vi "Calibration-LineN-Acquisition.vi"(7 "Cal Line?":i32, 8 "error in (no error)":errorcluster, 11 "Calibration-RunTest in":refnum<class "Calibration-RunTest.lvclass">) -> (0 "error out":errorcluster, 3 "Calibration-RunTest out":refnum<class "Calibration-RunTest.lvclass">)   [LabVIEW 2014, in "Calibration-RunTest.lvclass"]
uses:
  Calibration-RunTest.lvclass
  Reuse Library/Keyence LK-G5000/Public/enum/LKIF_OUTNO.ctl
  Reuse Library/Keyence LK-G5000/Keyence LK-G5000.lvlib
  Motion Control/Motion-ControlAll.lvclass
panel:
  out "Raw Cal Data":dbl[](array[numeric])
  out "Laser Value":sgl format="%_6g"
  out "stop collecting":bool=TRUE
  out "Meas 1 Dyn Data":dbl[](graph)
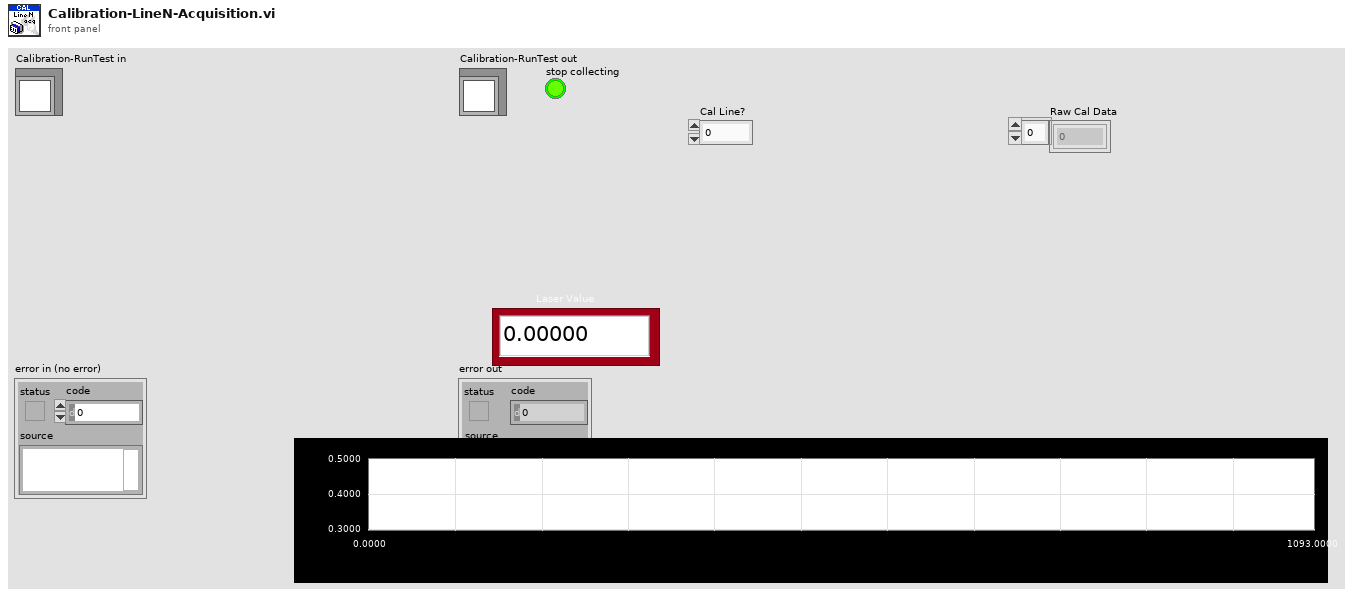
[diagram p1: front panel]
types:
  T1 = typedef "Keyence LK-G5000.lvlib/LKIF_OUTNO.ctl" = i32
  T2 = typedef "Keyence LK-G5000.lvlib/LKIF_FLOATRESULT.ctl" = i32
  T3 = cluster{"OutNo":i32, "LKIF_FLOATRESULT":T2, "Value":sgl}[]
  T4 = cluster{"OutNo":i32, "LKIF_FLOATRESULT":T2, "Value":sgl}
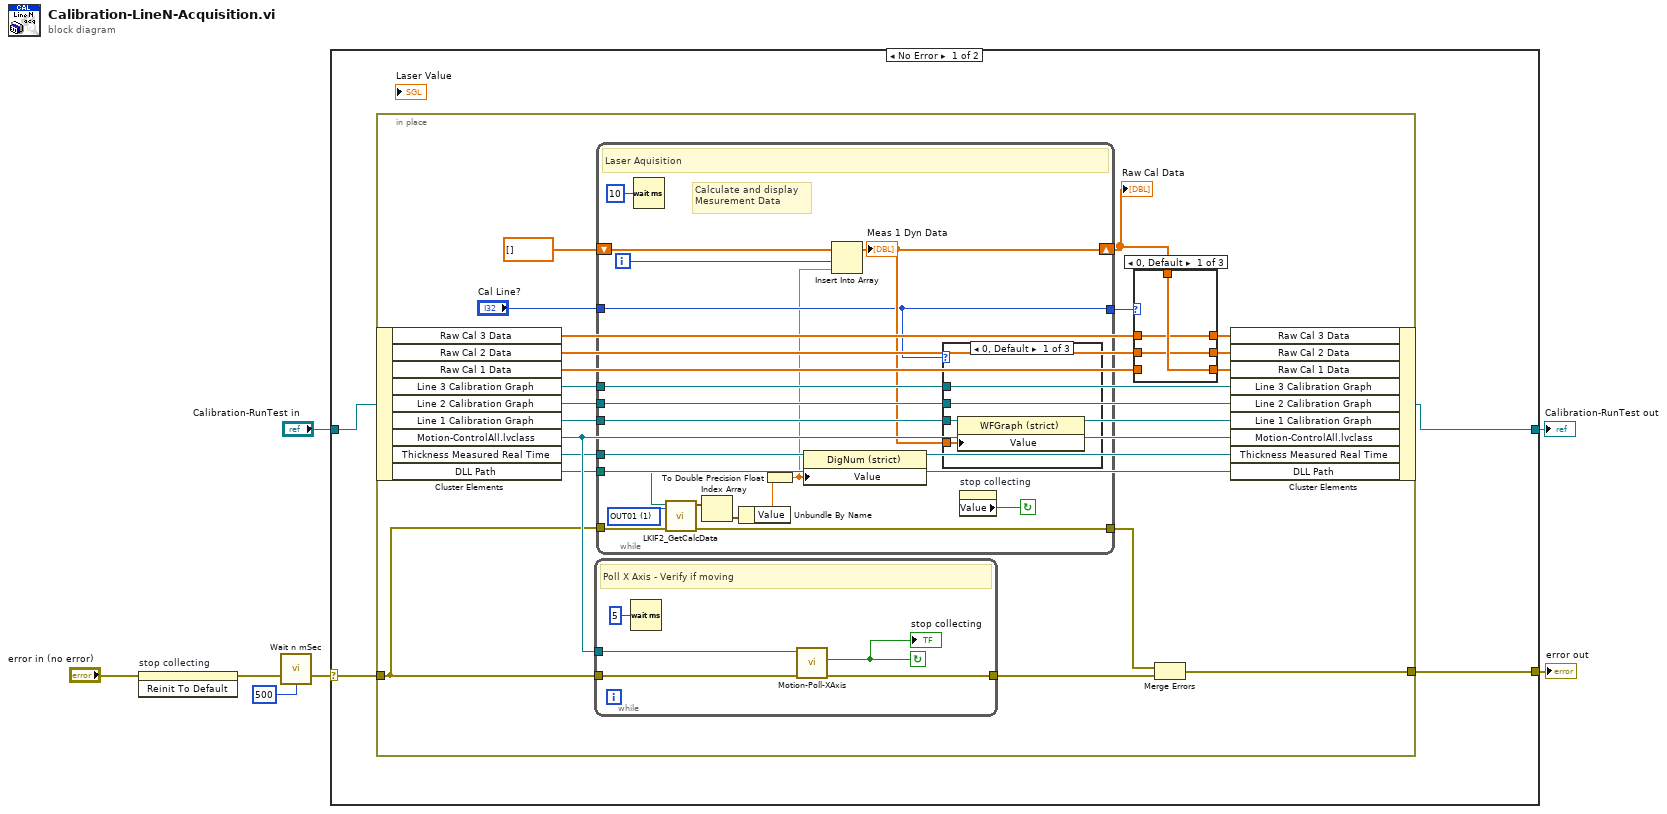
[diagram p0: block diagram]
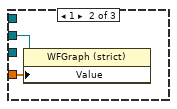
[diagram p4: hidden frame]
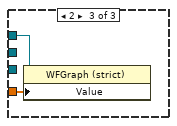
[diagram p5: hidden frame]
diagram:
  n1 = invoke on="stop collecting" class="Bool (strict)" method="Reinit To Default"(error in="error in (no error)") -> (error out=w1:errorcluster)  [unwired: 2 in, 2 out]
  n2 = call <vilib>:"Wait n mSec.vi"("error in (no error)"=w1, "Milliseconds to Wait (500)"=u32 500) -> ("error out"=w2:errorcluster)  [unwired: 13 in]
  n3 = case shown="No Error" w2 {
    selector: w2 -> [w10 w71]
    tunnel: [w9 w71] -> w7
    tunnel: [w8 w70] -> w5
    tunnel: "Calibration-RunTest in" -> [w11 w70]
    frame No Error {
      n4 = in-place {
        in-place-border: w10 -> [w12]
        in-place-border: [w29] -> w9
        n5 = in-place-cluster #1(w11) -> ("Raw Cal 3 Data"=w17:dbl[], "Raw Cal 2 Data"=w19:dbl[], "Raw Cal 1 Data"=w20:dbl[], "Line 3 Calibration Graph"=w25:refnum<vi>, "Line 2 Calibration Graph"=w26:refnum<vi>, "Line 1 Calibration Graph"=w27:refnum<vi>, "Motion-ControlAll.lvclass"=w28:refnum<class "Motion-ControlAll.lvclass">, "Thickness Measured Real Time"=w14:refnum<vi>, "DLL Path"=w13:path)
        n6 = while {
          tunnel: w12 -> [w44]
          tunnel: [w42] -> w31
          tunnel: w28 -> [w43]
          stop <- w41 continue-if-true
          # "Poll X Axis - Verify if moving"
          n7 = Wait (ms)(milliseconds to wait=u32 5) -> ()  [unwired: 1 out]
          n8 = call "Motion-Poll-XAxis.vi"("error in (no error)"=w44, "Motion-ControlAll in"=w43) -> ("error out"=w42:errorcluster, "X axis \nstopped"=w41:bool)  [unwired: 7 in, 1 out]
          "stop collecting" <- w41
        }
        n9 = while {
          tunnel: w12 -> [w63]
          tunnel: [w59] -> w30
          shift-right: [w53] -> w22
          shift-left: dbl[] [] -> [w57]
          tunnel: w27 -> [w54]
          tunnel: w26 -> [w52]
          tunnel: w25 -> [w51]
          tunnel: "Cal Line?" -> [w50]
          tunnel: [w50] -> w23
          tunnel: w14 -> [w49]
          tunnel: w13 -> [w46]
          i -> [w56]
          stop <- w55 continue-if-true
          w62 = T1 1 items=["OUT01"=1, "OUT02"=2, "OUT03"=4, "OUT04"=8, "OUT05"=16, "OUT06"=32, "OUT07"=64, "OUT08"=128, "OUT09"=256, "OUT10"=512, "OUT11"=1024, "OUT12"=2048, "ALL OUT"=4095] ("OutNo (OUT1)")
          # "Calculate and display \nMesurement Data"
          # "Laser Aquisition"
          n10 = Wait (ms)(milliseconds to wait=u32 10) -> ()  [unwired: 1 out]
          n11 = call "LKIF2_GetCalcData.vi"("OutNo (OUT1)"=w62, "error in (no error)"=w63, "path in"=w46) -> ("error out"=w59:errorcluster, "CalcData"=w61:T3)  [unwired: 7 in]
          n12 = Index Array(array=w61) -> (element=w60:T4)  [unwired: 1 in]
          n13 = Unbundle By Name(w60) -> ("Value"=w48:sgl)
          n14 = To Double Precision Float(number=w48) -> (double precision float=w47:dbl)
          n15 = property class="DigNum (strict)"(reference=w49, "Value"=w47) -> ()  [unwired: 1 in, 2 out]
          n16 = Insert Into Array(array=w57, index=w56, new element=w47) -> (w53:dbl[])
          "Meas 1 Dyn Data" <- w53
          n17 = case shown="0, Default" w50 {
            tunnel: w54 -> [w65 _ _]
            tunnel: w53 -> [w64 w66 w69]
            tunnel: w52 -> [_ w67 _]
            tunnel: w51 -> [_ _ w68]
            frame 0, Default {
              n18 = property class="WFGraph (strict)"(reference=w65, "Value"=w64) -> ()  [unwired: 1 in, 2 out]
            }
            frame 1 {
              n19 = property class="WFGraph (strict)"(reference=w67, "Value"=w66) -> ()  [unwired: 1 in, 2 out]
            }
            frame 2 {
              n20 = property class="WFGraph (strict)"(reference=w68, "Value"=w69) -> ()  [unwired: 1 in, 2 out]
            }
          }
          n21 = property on="stop collecting" class="Bool (strict)"() -> ("Value"=w55:bool)  [unwired: 2 in, 2 out]
        }
        "Raw Cal Data" <- w22
        n22 = case shown="0, Default" w23 {
          tunnel: [w34 w37 w40] -> w21
          tunnel: w22 -> [w34 w36 w38]
          tunnel: w20 -> [_ w37 w40]
          tunnel: w19 -> [w33 _ w39]
          tunnel: [w33 w36 w39] -> w18
          tunnel: w17 -> [w32 w35 _]
          tunnel: [w32 w35 w38] -> w16
          frame 0, Default {
          }
          frame 1 {
          }
          frame 2 {
          }
        }
        n23 = Merge Errors(w30, w31) -> (w29:errorcluster)
        n24 = in-place-cluster #1("Raw Cal 3 Data"=w16, "Raw Cal 2 Data"=w18, "Raw Cal 1 Data"=w21, "Line 3 Calibration Graph"=w25, "Line 2 Calibration Graph"=w26, "Line 1 Calibration Graph"=w27, "Motion-ControlAll.lvclass"=w28, "Thickness Measured Real Time"=w14, "DLL Path"=w13) -> (w8:refnum<class "Calibration-RunTest.lvclass">)
      }
    }
    frame Error {
    }
  }
  "error out" <- w7
  "Calibration-RunTest out" <- w5
